vi "LaunchDelRx.vi"(8 "error in (no error)":errorcluster, 10 "milliseconds to wait":u32, 11 "Module ID":i32) -> (0 "error out":errorcluster)   [LabVIEW 2015, in "Serializer.lvlib"]
uses:
  Serializer.lvlib
  DelayedRX.vi
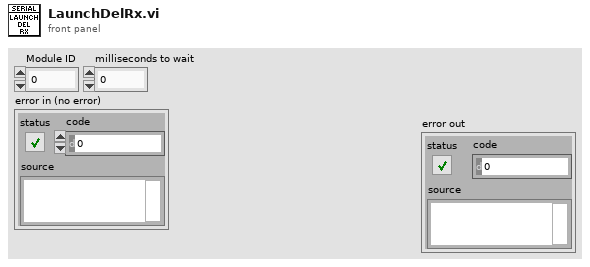
[diagram p1: front panel]
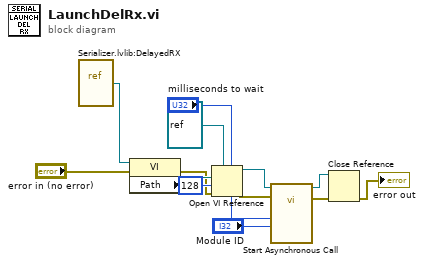
[diagram p0: block diagram]
diagram:
  n1 = vi-ref "Serializer.lvlib:DelayedRX.vi"() -> (w13:refnum<vi>)
  n2 = property class="VI"(reference=w13, error in="error in (no error)") -> (error out=w2:errorcluster, "Path"=w12:path)  [unwired: 1 out]
  n3 = Open VI Reference(type specifier VI Refnum (for type only)=refnum<vi> refnum, vi path=w12, options=128, error in (no error)=w2) -> (vi reference=w10:refnum<vi>, error out=w9:errorcluster)  [unwired: 2 in]
  n4 = call-by-ref "Start Asynchronous Call"(reference=w10, error in=w9, "Module ID"="Module ID", "milliseconds to wait"="milliseconds to wait") -> (reference out=w4:refnum<vi>, error out=w5:errorcluster)  [unwired: 10 in]
  n5 = Close Reference(reference=w4, error in (no error)=w5) -> (error out=→"error out":errorcluster)
